vi "Replace 2D array in default JSON.vi"(8 "error in (no error)":errorcluster, 11 "VCluster with Array of Arrays":variant=variant(cluster{"InitialCluster":cluster{"Array":variant[]}} {"InitialCluster"={"Array"=[variant(cluster{"Name":string, "Dept":string, "2DArray":variant[]} {"Name"="S.Raakesh", "Dept"="E", "2DArray"=[variant(variant[] [variant(u64 1), variant(u64 2)]), variant(variant[] [variant(u64 3), variant(u64 4)])]}), variant(cluster{"Name":string, "Dept":string, "2DArray":variant[]} {"Name"="1ABC2", "Dept"="E", "2DArray"=[variant(variant[] [variant(u64 1), variant(u64 2)]), variant(variant[] [variant(u64 3), variant(u64 4)])]})]}})) -> (0 "error out":errorcluster, 3 "VCluster with replaced 2D Array":variant)   [LabVIEW 2015]
uses:
  <vilib>/Utility/Data Type/NI_Data Type.lvlib
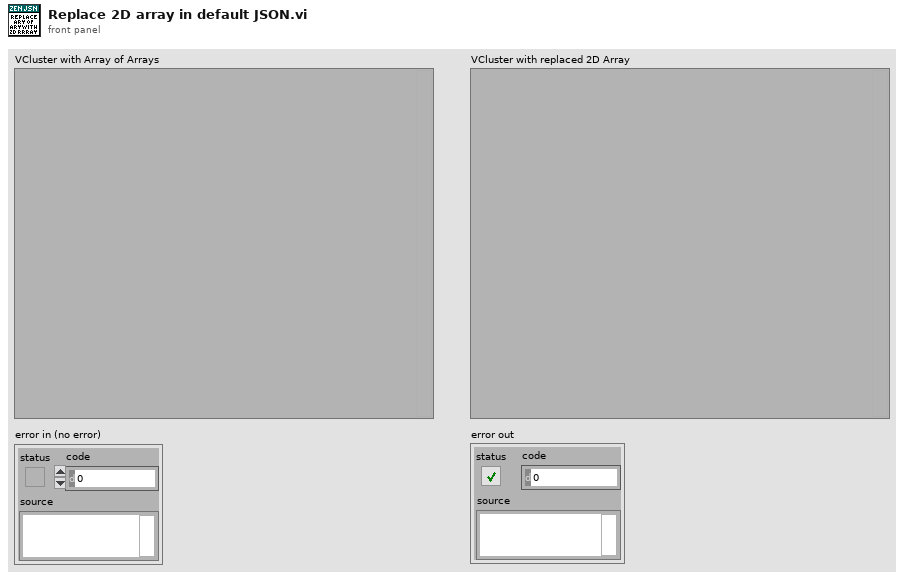
[diagram p1: front panel]
types:
  T1 = typedef "NI_Data Type.lvlib/Data Type.ctl" = enum8{"Invalid Type", "Void", "I8", "I16", "I32", "I64", "U8", "U16", "U32", "U64", "Single Float", "Double Float", "Extended Float", "Single Complex", "Double Complex", "Extended Complex", "Enum U8", "Enum U16", "Enum U32", "Enum U64", "Single Float With Unit", "Double Float With Unit", "Extended Float With Unit", "Single Complex with Unit", "Double Complex with Unit", "Extended Complex with Unit", "Boolean", "String", "Path", "Picture", "Tag", "Array", "Cluster", "Variant", "LV Variant", "Waveform", "Timestamp", "Digital Waveform", "Digital Data", "ExpressData", "Refnum", "External Data", "VI", "Poly VI", "LabVIEW Class Instance", "Fixed Point"}
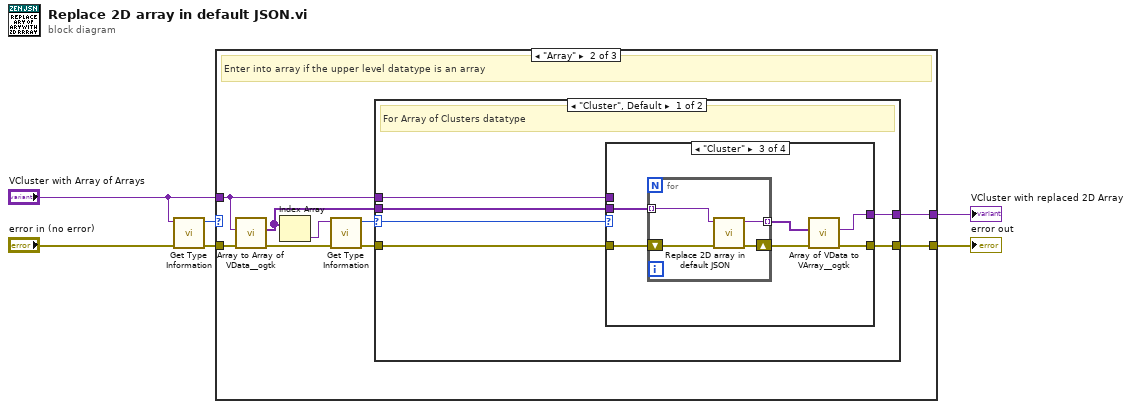
[diagram p0: block diagram]
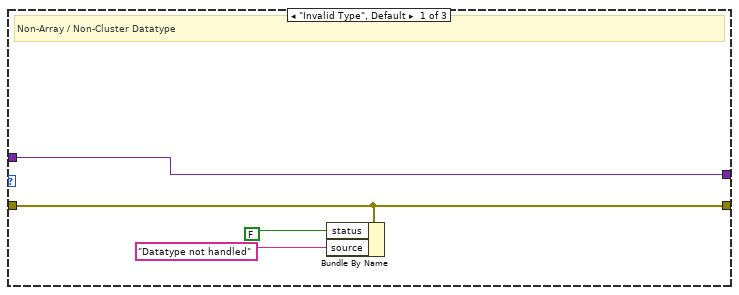
[diagram p2: hidden frame]
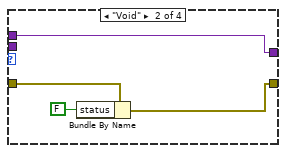
[diagram p4: hidden frame]
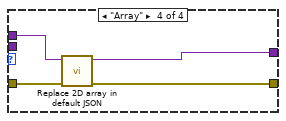
[diagram p5: hidden frame]
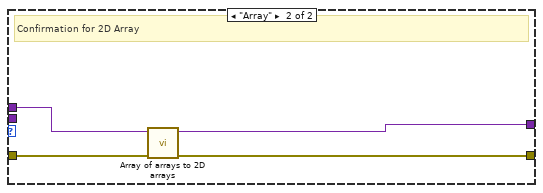
[diagram p6: hidden frame]
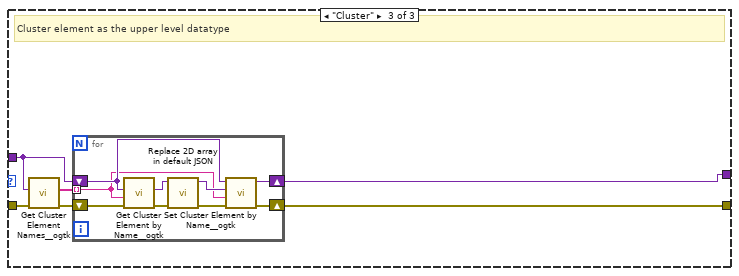
[diagram p7: hidden frame]
diagram:
  n1 = call <vilib>:"Get Type Information.vi"("error in (no error)"="error in (no error)", "Variant"="VCluster with Array of Arrays") -> ("error out"=w5:errorcluster, "Type"=w6:T1)  [unwired: 5 in, 3 out]
  n2 = case shown="\"Array\"" w6 {
    tunnel: "VCluster with Array of Arrays" -> [w10 w17 w54]
    tunnel: w5 -> [w7 w15 w53]
    tunnel: [w10 w18 w51] -> w3
    tunnel: [w7 w19 w50] -> w2
    frame "Invalid Type", Default {
      # "Non-Array / Non-Cluster Datatype"
      n3 = Bundle By Name(cluster=w7, "status"=FALSE, "source"="Datatype not handled") -> ()  [unwired: 1 out]
    }
    frame "Array" {
      # "Enter into array if the upper level datatype is an array"
      n4 = call <userlib>:"Array to Array of VData__ogtk.vi"("error in (no error)"=w15, "MultiD Array"=w17) -> ("error out"=w14:errorcluster, "1D Array of Variants"=w12:variant[])  [unwired: 8 in]
      n5 = Index Array(array=w12) -> (element=w11:variant)  [unwired: 1 in]
      n6 = call <vilib>:"Get Type Information.vi"("error in (no error)"=w14, "Variant"=w11) -> ("error out"=w13:errorcluster, "Type"=w16:T1)  [unwired: 5 in, 3 out]
      n7 = case shown="\"Cluster\", Default" w16 {
        selector: w16 -> [w21 _]
        tunnel: w13 -> [w22 w48]
        tunnel: [w25 w46] -> w19
        tunnel: [w24 w49] -> w18
        tunnel: w17 -> [w23 w47]
        tunnel: w12 -> [w20 _]
        frame "Cluster", Default {
          # "For Array of Clusters datatype"
          n8 = case shown="\"Cluster\"" w21 {
            tunnel: w20 -> [_ _ w37 _]
            tunnel: [w27 w31 w35 w44] -> w24
            tunnel: w23 -> [w27 w31 _ w45]
            tunnel: w22 -> [w26 w30 w34 w43]
            tunnel: [w26 w28 w32 w42] -> w25
            frame "Invalid Type", Default {
            }
            frame "Void" {
              n9 = Bundle By Name(cluster=w30, "status"=FALSE) -> (w28:errorcluster)
            }
            frame "Cluster" {
              n10 = for {
                tunnel: w37 -> [w41] mode=indexing
                tunnel: [w40] -> w36 mode=indexing
                shift-right: [w39] -> w33
                shift-left: w34 -> [w38]
                n11 = call "Replace 2D array in default JSON.vi"("error in (no error)"=w38, "VCluster with Array of Arrays"=w41) -> ("error out"=w39:errorcluster, "VCluster with replaced 2D Array"=w40:variant)  [unwired: 8 in]
              }
              n12 = call <userlib>:"Array of VData to VArray__ogtk.vi"("error in (no error)"=w33, "1D Array of VData"=w36) -> ("error out"=w32:errorcluster, "VArray"=w35:variant)  [unwired: 8 in]
            }
            frame "Array" {
              n13 = call "Replace 2D array in default JSON.vi"("error in (no error)"=w43, "VCluster with Array of Arrays"=w45) -> ("error out"=w42:errorcluster, "VCluster with replaced 2D Array"=w44:variant)  [unwired: 8 in]
            }
          }
        }
        frame "Array" {
          # "Confirmation for 2D Array"
          n14 = call "Array of arrays to 2D arrays.vi"("error in (no error)"=w48, "Variant in"=w47) -> ("error out"=w46:errorcluster, "Variant out"=w49:variant)  [unwired: 7 in, 1 out]
        }
      }
    }
    frame "Cluster" {
      # "Cluster element as the upper level datatype"
      n15 = call <userlib>:"Get Cluster Element Names__ogtk.vi"("error in (no error)"=w53, "Cluster"=w54) -> ("error out"=w52:errorcluster, "Element Names"=w55:string[])  [unwired: 8 in]
      n16 = for {
        tunnel: w55 -> [w57] mode=indexing
        shift-right: [w60] -> w50
        shift-left: w52 -> [w64]
        shift-right: [w56] -> w51
        shift-left: w54 -> [w58]
        n17 = call <userlib>:"Get Cluster Element by Name__ogtk.vi"("error in (no error)"=w64, "Element Name"=w57, "Cluster"=w58) -> ("error out"=w63:errorcluster, "VElement"=w62:variant)  [unwired: 6 in, 1 out]
        n18 = call "Replace 2D array in default JSON.vi"("error in (no error)"=w63, "VCluster with Array of Arrays"=w62) -> ("error out"=w61:errorcluster, "VCluster with replaced 2D Array"=w59:variant)  [unwired: 8 in]
        n19 = call <userlib>:"Set Cluster Element by Name__ogtk.vi"("error in (no error)"=w61, "Element Name (\"\": New Element Data Name)"=w57, "New Element Value"=w59, "Cluster"=w58) -> ("error out"=w60:errorcluster, "VCluster out"=w56:variant)  [unwired: 5 in, 1 out]
      }
    }
  }
  "VCluster with replaced 2D Array" <- w3
  "error out" <- w2
